vi "Tag Change Value.vi"(10 "Data":variant, 11 "IFD_Tag in":refnum<class "IFD_Tag.lvclass">) -> (3 "IFD_Tag out":refnum<class "IFD_Tag.lvclass">)   [LabVIEW 2016, in "IFD_Tag.lvclass"]
uses:
  IFD_Tag.lvclass
  IFD_Tag.lvclass/IFD_Tag.ctl
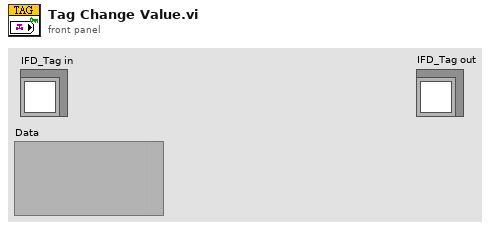
[diagram p1: front panel]
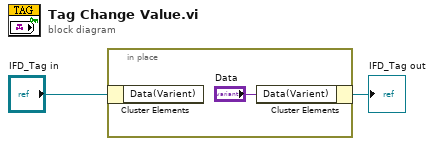
[diagram p0: block diagram]
diagram:
  n1 = in-place {
    n2 = in-place-cluster #1("IFD_Tag in") -> ()  [unwired: 1 out]
    n3 = in-place-cluster #1("Data(Varient)"="Data") -> (→"IFD_Tag out":refnum<class "IFD_Tag.lvclass">)
  }
